vi "test metadata.vi"() -> ()   [LabVIEW 2014, in "NISE_CEF_Tests.lvlib"]
uses:
  NISE_CEF_Tests.lvlib
  Trunk/Configuration Framework/serializable configuration/NISE_CEF_serializable configuration.lvclass
panel:
  out "overwriteok":bool
  out "setgetok":bool
  out "deletedok":bool
  out "ook":errorcluster
  out "error 538311":errorcluster
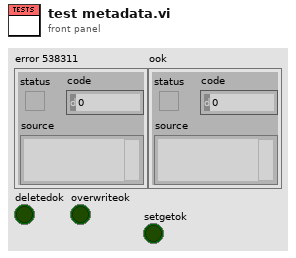
[diagram p1: front panel]
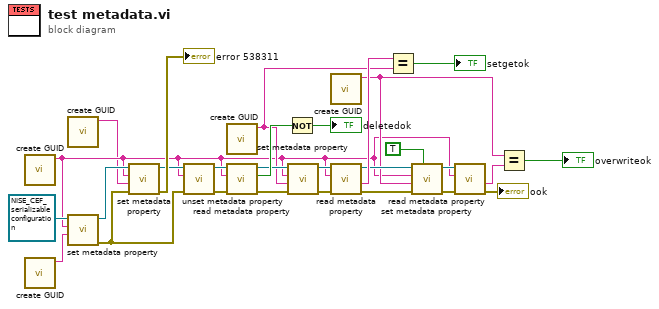
[diagram p0: block diagram]
diagram:
  n1 = call "create GUID.vi"() -> ("uuid"=w3:string)  [unwired: 10 in, 1 out]
  n2 = call "create GUID.vi"() -> ("uuid"=w2:string)  [unwired: 10 in, 1 out]
  n3 = call "create GUID.vi"() -> ("uuid"=w1:string)  [unwired: 10 in, 1 out]
  n4 = call "set metadata property.vi"("value"=w2, "key"=w3, "configuration in"=refnum<class "NISE_CEF_serializable configuration.lvclass"> refnum ("configuration")) -> ("error out"=w25:errorcluster, "configuration out"=w28:refnum<class "NISE_CEF_serializable configuration.lvclass">)  [unwired: 7 in]
  n5 = call "set metadata property.vi"("error in"=w25, "value"=w1, "key"=w3, "configuration in"=w28) -> ("error out"=→"error 538311":errorcluster, "configuration out"=w26:refnum<class "NISE_CEF_serializable configuration.lvclass">)  [unwired: 6 in]
  n6 = call "unset metadata property.vi"("error in"=w25, "key"=w3, "configuration in"=w26) -> ("error out"=w24:errorcluster, "configuration out"=w23:refnum<class "NISE_CEF_serializable configuration.lvclass">)  [unwired: 7 in]
  n7 = call "create GUID.vi"() -> ("uuid"=w16:string)  [unwired: 10 in, 1 out]
  n8 = call "read metadata property.vi"("error in"=w24, "key"=w3, "configuration in"=w23) -> ("error out"=w21:errorcluster, "found"=w22:bool, "configuration out"=w20:refnum<class "NISE_CEF_serializable configuration.lvclass">)  [unwired: 5 in, 1 out]
  n9 = Not(x=w22) -> (.not. x?=→"deletedok":bool)
  n10 = call "set metadata property.vi"("error in"=w21, "value"=w16, "key"=w3, "configuration in"=w20) -> ("error out"=w19:errorcluster, "configuration out"=w18:refnum<class "NISE_CEF_serializable configuration.lvclass">)  [unwired: 6 in]
  n11 = call "create GUID.vi"() -> ("uuid"=w4:string)  [unwired: 10 in, 1 out]
  n12 = call "read metadata property.vi"("error in"=w19, "key"=w3, "configuration in"=w18) -> ("error out"=w13:errorcluster, "value"=w17:string, "configuration out"=w12:refnum<class "NISE_CEF_serializable configuration.lvclass">)  [unwired: 5 in, 1 out]
  n13 = Equal?(x=w17, y=w16) -> (x = y?=→"setgetok":bool)
  n14 = call "set metadata property.vi"("overwrite?"=TRUE, "error in"=w13, "value"=w4, "key"=w3, "configuration in"=w12) -> ("error out"=w9:errorcluster, "configuration out"=w10:refnum<class "NISE_CEF_serializable configuration.lvclass">)  [unwired: 5 in]
  n15 = call "read metadata property.vi"("error in"=w9, "key"=w3, "configuration in"=w10) -> ("error out"=→"ook":errorcluster, "value"=w7:string)  [unwired: 5 in, 2 out]
  n16 = Equal?(x=w4, y=w7) -> (x = y?=→"overwriteok":bool)
